vi "fgv_Bcknd Imaging window status.vi"(8 "error in (no error)":errorcluster, 9 "Function":T1, 11 "Background MovCor window is open":bool) -> (0 "error out":errorcluster, 3 "Background MovCor window is open":bool)   [LabVIEW 2017]
uses:
  Typedefs/Read Write Enum.ctl
  General Globals.vi
panel:
  # "SUBROUTINE"
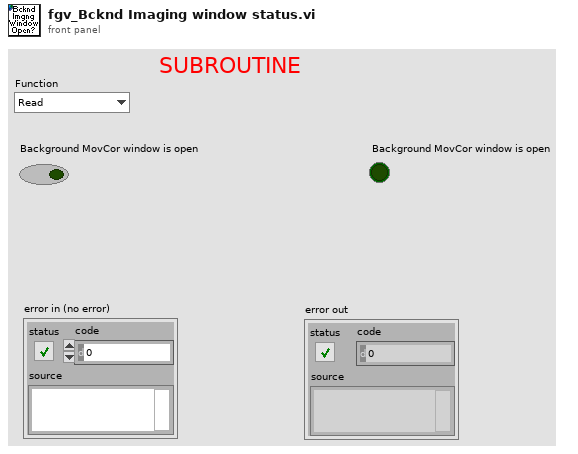
[diagram p1: front panel]
types:
  T1 = typedef "Read Write Enum.ctl" = enum16{"Read", "Write"}
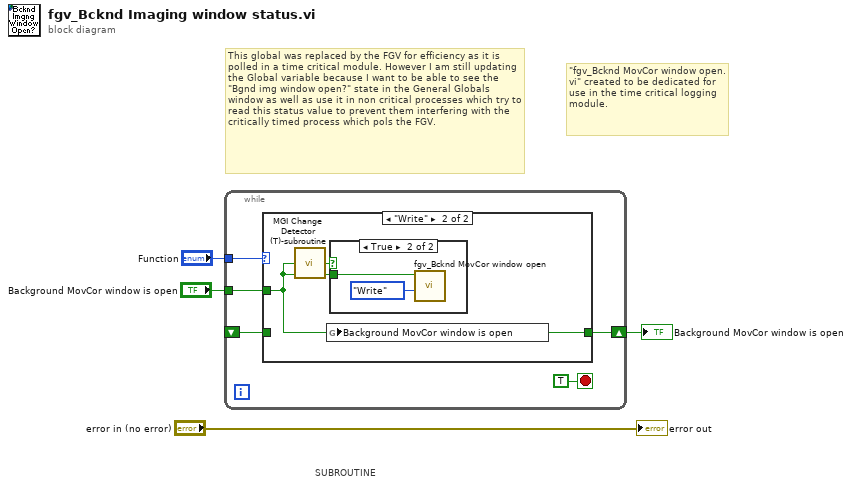
[diagram p0: block diagram]
diagram:
  # "\"fgv_Bcknd MovCor window open.vi\" created to be dedicated for use in the time critical logging module."
  # "This global was replaced by the FGV for efficiency as it is polled in a time critical module. However I am still updating the Global variable because I want to be able to see the \"Bgnd img window open?\" state in the General Globals window as well as use it in non critical processes which try to read this status value to prevent them interfering with the critically timed process which pols the FGV."
  # "SUBROUTINE"
  n1 = while {
    tunnel: "Function" -> [w8]
    tunnel: "Background MovCor window is open" -> [w7]
    shift-right: [w6] -> w2
    shift-left: _ -> [w5]
    stop <- TRUE stop-if-true
    n2 = case shown="\"Write\"" w8 {
      tunnel: w7 -> [_ w11]
      tunnel: [w10 w11] -> w6
      tunnel: w5 -> [w10 _]
      frame "Read", Default {
      }
      frame "Write" {
        n3 = call "MGI Change Detector (T)-subroutine.vi"("Value"=w11) -> ("Changed?"=w12:bool)
        n4 = global write "General Globals.vi" "Background MovCor window is open"(w11) -> ()
        n5 = case shown="True" w12 {
          tunnel: w11 -> [_ w14]
          frame False {
          }
          frame True {
            n6 = call "fgv_Bcknd MovCor window open.vi"("Function"=Read_Write_Enum."Write", "Background MovCor window is open"=w14) -> ()  [unwired: 8 in, 2 out]
          }
        }
      }
    }
  }
  "Background MovCor window is open" <- w2
  "error out" <- "error in (no error)"
